vi "Write DO with model.vi"(7 "Device model":string, 8 "error in":errorcluster, 10 "Motor control":T1={"EN1"=FALSE, "DIR1"=TRUE, "EN2"=FALSE, "DIR2"=TRUE, "TOG"=FALSE}, 11 "Module ID":i32=-1) -> (0 "error out":errorcluster)   [LabVIEW 2020]
doc: "Writes DO to DAQ device dependant on the DAQ model."
uses:
  NI_DAQ/Libraries/NI DAQ/NI DAQ.lvlib
  Controls/Motor controls---typedef.ctl
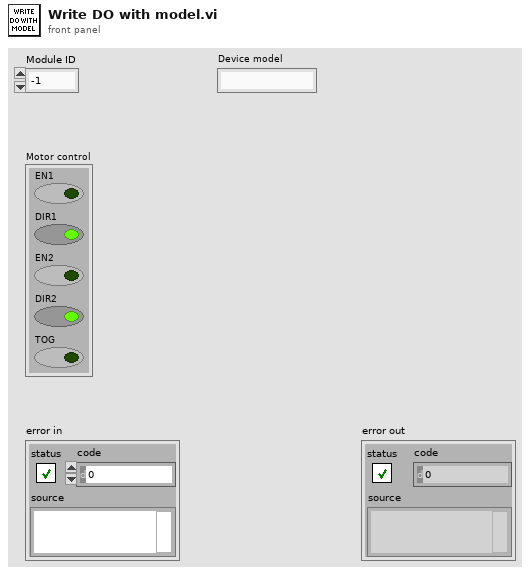
[diagram p1: front panel]
types:
  T1 = typedef "Motor controls---typedef.ctl" = cluster{"EN1":bool, "DIR1":bool, "EN2":bool, "DIR2":bool, "TOG":bool}
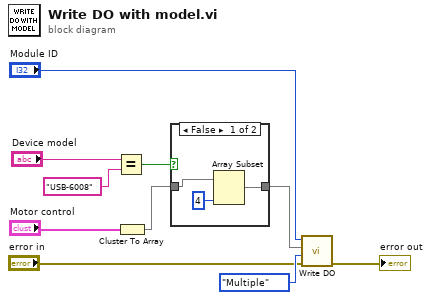
[diagram p0: block diagram]
diagram:
  n1 = Equal?(x="Device model", y="USB-6008") -> (x = y?=w5:bool)
  n2 = Cluster To Array(cluster="Motor control") -> (array=w2:bool[])
  n3 = case shown="False" w5 {
    tunnel: w2 -> [w12 w14]
    tunnel: [w11 w14] -> w1
    frame False {
      n4 = Array Subset(array=w12, length=4) -> (w11:bool[])  [unwired: 1 in]
    }
    frame True {
    }
  }
  n5 = call "Write DO.vi"("error in"="error in", "Samples"=enum16{"Single", "Multiple"}."Multiple", "Data"=w1, "Module ID"="Module ID") -> ("error out"=→"error out":errorcluster)  [unwired: 7 in]
